vi "Set Measurement Count.vi"(8 "error in (no error)":errorcluster, 10 "Measurement Count":i32=1 min=1 max=300000 step=1, 11 "VISA resource name":refnum<visa-resource-name>="USB0::0x05E6::0x2461::04090181::INSTR") -> (0 "error out":errorcluster, 3 "VISA resource name out":refnum<visa-resource-name>="USB0::0x05E6::0x2461::04090181::INSTR")   [LabVIEW 2022 SP3, in "Keithley 2450.lvlib"]
doc: "This sets the number of measurements to be performed when a measurement is requested."
uses:
  Keithley 2450.lvlib
panel:
  in  "Digitizer (False)":bool
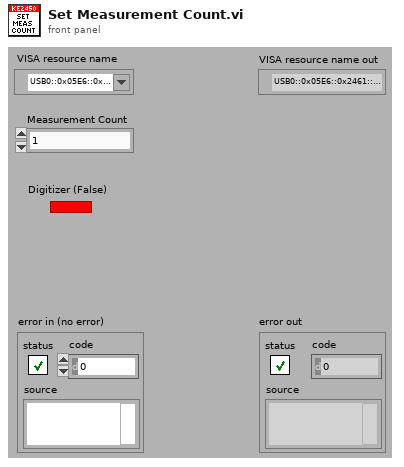
[diagram p1: front panel]
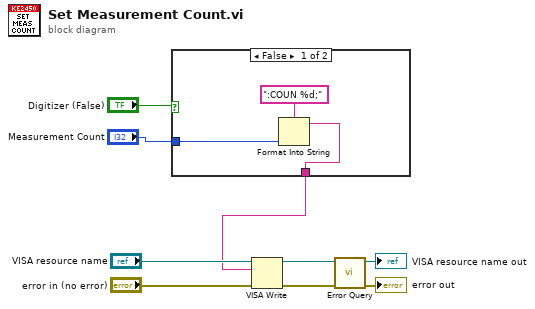
[diagram p0: block diagram]
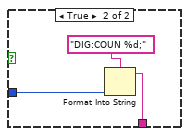
[diagram p2: hidden frame]
diagram:
  n1 = case shown="False" "Digitizer (False)" {
    tunnel: "Measurement Count" -> [w11 w14]
    tunnel: [w10 w13] -> w1
    frame False {
      n2 = Format Into String(format string=":COUN %d;", w11) -> (resulting string=w10:string)  [unwired: 2 in, 1 out]
    }
    frame True {
      n3 = Format Into String(format string="DIG:COUN %d;", w14) -> (resulting string=w13:string)  [unwired: 2 in, 1 out]
    }
  }
  n4 = VISA Write(VISA resource name="VISA resource name", write buffer=w1, error in (no error)="error in (no error)") -> (VISA resource name out=w5:refnum<visa-resource-name>, error out=w4:errorcluster)  [unwired: 1 out]
  n5 = call "Error Query.vi"("error in (no error)"=w4, "VISA resource name"=w5) -> ("error out"=→"error out":errorcluster, "VISA resource name out"=→"VISA resource name out":refnum<visa-resource-name>)  [unwired: 8 out]
